vi "Getpinstatusresponse.vi"(8 "error in (no error)":errorcluster, 11 "Serial Device in":refnum<class "Serial Device.lvclass">) -> (0 "error out":errorcluster, 2 "Value":string, 3 "Serial Device out":refnum<class "Serial Device.lvclass">)   [LabVIEW 2019, in "Serial Device.lvclass"]
doc: "Este Vi se encarag de leer del micro los valores del los pines seleccionados. Eventualmente son mostrados en el interfaz"
uses:
  Serial Device.lvclass
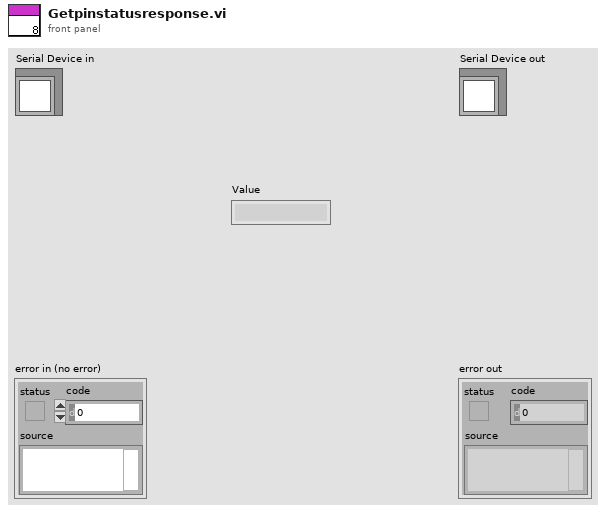
[diagram p1: front panel]
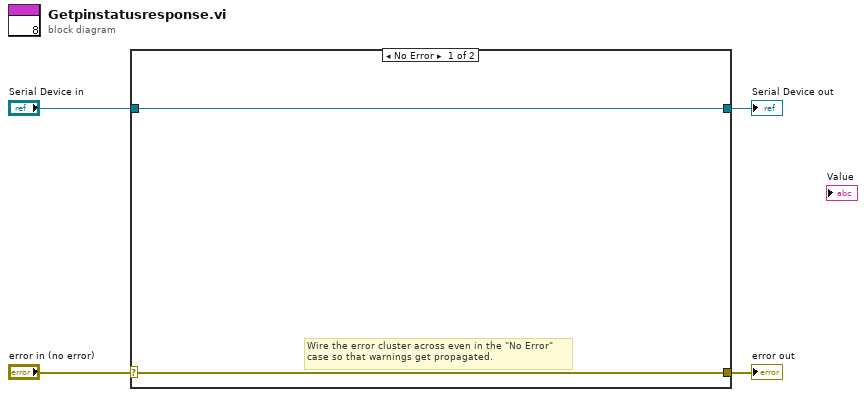
[diagram p0: block diagram]
diagram:
  n1 = case shown="No Error" "error in (no error)" {
    selector: "error in (no error)" -> [w5 w8]
    tunnel: [w5 w8] -> w3
    tunnel: [w6 w7] -> w1
    tunnel: "Serial Device in" -> [w6 w7]
    frame No Error {
      # "Wire the error cluster across even in the \"No Error\"\ncase so that warnings get propagated."
    }
    frame Error {
    }
  }
  "error out" <- w3
  "Serial Device out" <- w1
